vi "Driver VISA Query.vi"(4 "End Symble":u16(ring)=1 items=["None", "\\n", "\\r\\n"], 6 "Read Length":u32=1024, 7 "Read?":bool, 8 "error in (no error)":errorcluster, 9 "Timeout":u32=100, 10 "buffer in":string, 11 "VISA resource name":refnum<visa-resource-name>) -> (0 "error out":errorcluster, 2 "buffer out":string, 3 "VISA resource name out":refnum<visa-resource-name>)   [LabVIEW 2020]
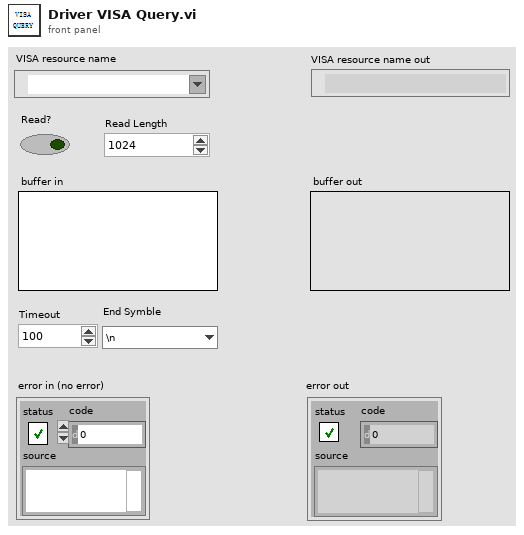
[diagram p1: front panel]
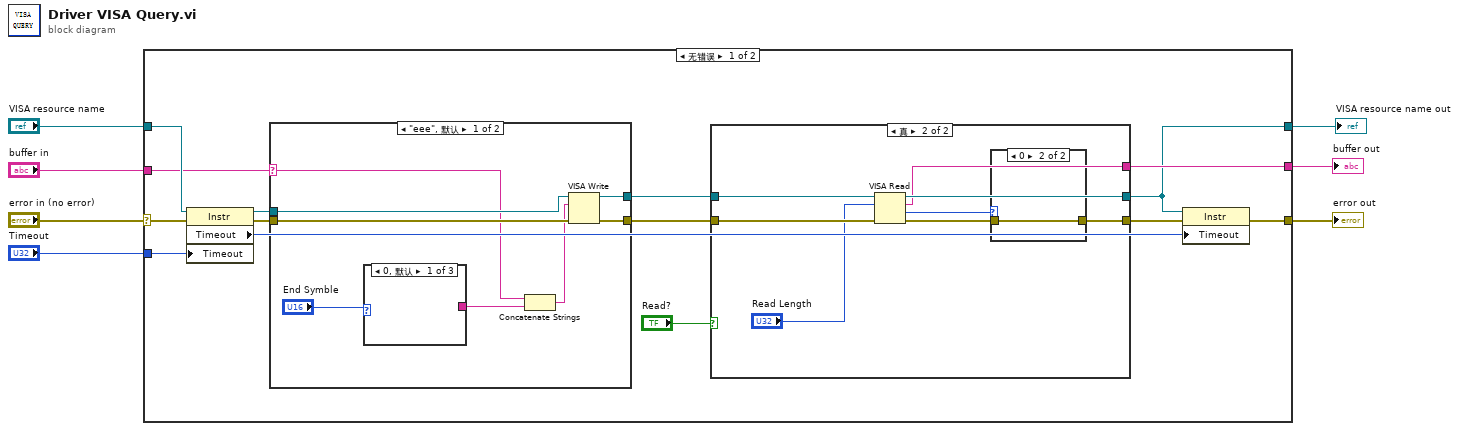
[diagram p0: block diagram]
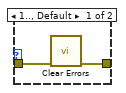
[diagram p3: hidden frame]
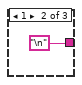
[diagram p4: hidden frame]
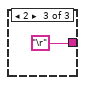
[diagram p5: hidden frame]
diagram:
  n1 = case shown="无错误" "error in (no error)" {
    selector: "error in (no error)" -> [w17 w47]
    tunnel: "VISA resource name" -> [w20 w48]
    tunnel: [w19 _] -> w6
    tunnel: [w13 w48] -> w4
    tunnel: [w10 w47] -> w3
    tunnel: "buffer in" -> [w9 _]
    tunnel: "Timeout" -> [w8 _]
    frame No Error {
      n2 = property class="Instr"(reference=w20, error in=w17, "Timeout"=w8) -> (reference out=w18:refnum<visa-resource-name>, error out=w16:errorcluster, "Timeout"=w12:u32)
      n3 = case shown="\"eee\", 默认" w9 {
        selector: w9 -> [w37 _]
        tunnel: [w42 w46] -> w21
        tunnel: w18 -> [w41 w46]
        tunnel: w16 -> [w40 w45]
        tunnel: [w39 w45] -> w15
        frame "eee", Default {
          n4 = case shown="0, 默认" "End Symble" {
            tunnel: [_ "\n" "\r"] -> w36
            frame 0, Default {
            }
            frame 1 {
            }
            frame 2 {
            }
          }
          n5 = Concatenate Strings(w37, w36) -> (w35:string)
          n6 = VISA Write(VISA resource name=w41, write buffer=w35, error in (no error)=w40) -> (VISA resource name out=w42:refnum<visa-resource-name>, error out=w39:errorcluster)  [unwired: 1 out]
        }
        frame "" {
        }
      }
      n7 = case shown="真" "Read?" {
        tunnel: [w23 w28] -> w13
        tunnel: [w22 w29] -> w11
        tunnel: w21 -> [w23 w31]
        tunnel: [_ w24] -> w19
        tunnel: w15 -> [w22 w30]
        frame False {
        }
        frame True {
          n8 = VISA Read(VISA resource name=w31, byte count="Read Length", error in (no error)=w30) -> (VISA resource name out=w28:refnum<visa-resource-name>, read buffer=w24:string, return count=w25:u32, error out=w27:errorcluster)
          n9 = case shown="0" w25 {
            tunnel: [w33 w34] -> w29
            tunnel: w27 -> [w32 w34]
            frame 1.., Default {
              n10 = call <vilib>:"Clear Errors.vi"("error in (no error)"=w32) -> ("error out"=w33:errorcluster)  [unwired: 5 in, 1 out]
            }
            frame 0 {
            }
          }
        }
      }
      n11 = property class="Instr"(reference=w13, error in=w11, "Timeout"=w12) -> (error out=w10:errorcluster)  [unwired: 1 out]
    }
    frame Error {
    }
  }
  "VISA resource name out" <- w4
  "error out" <- w3
  "buffer out" <- w6
